vi "sc5511a_spf_select_devices.vi"(5 "error in (no error)":errorcluster) -> (14 "Selected Resource":string, 19 "error out":errorcluster)   [LabVIEW 2010]
panel:
  in  "Cancel Button 2":bool
  in  "OK Button 2":bool
  out "source":string="No Ports  Found."
  in  "Resource Name":u16(ring) items=["COM1"]
  # "Please select a device from the pull-down menu:"
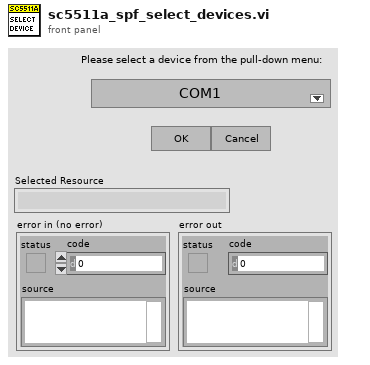
[diagram p1: front panel]
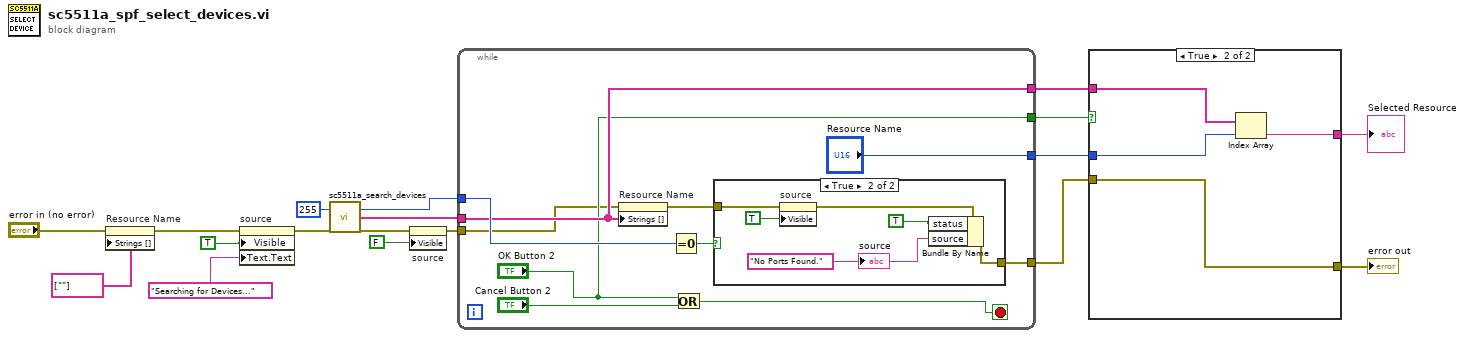
[diagram p0: block diagram]
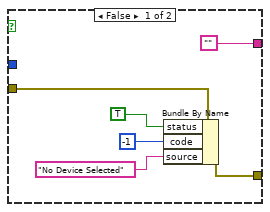
[diagram p2: hidden frame]
diagram:
  n1 = property on="Resource Name" class="Ring (strict)"(error in="error in (no error)", "Strings []"=string[] [""]) -> (error out=w10:errorcluster)  [unwired: 1 in, 1 out]
  n2 = property on="source" class="Str"(error in=w10, "Visible"=TRUE, "Text.Text"="Searching for Devices...") -> (error out=w8:errorcluster)  [unwired: 1 in, 1 out]
  n3 = call "sc5511a_search_devices.vi"("Devices to Search"=u32 255, "error in (no error)"=w8) -> ("Devices Found"=w7:u32, "Port_Name"=w6:string[], "error out"=w4:errorcluster)  [unwired: 15 in]
  n4 = property on="source" class="Str"(error in=w4, "Visible"=FALSE) -> (error out=w3:errorcluster)  [unwired: 1 in, 1 out]
  n5 = while {
    tunnel: ["Resource Name"] -> w17
    tunnel: [w22] -> w18
    tunnel: ["OK Button 2"] -> w16
    tunnel: w3 -> [w19]
    tunnel: [w25] -> w12
    tunnel: w7 -> [w23]
    tunnel: w6 -> [w22]
    stop <- w24 stop-if-true
    n6 = property on="Resource Name" class="Ring (strict)"(error in=w19, "Strings []"=w22) -> (error out=w26:errorcluster)  [unwired: 1 in, 1 out]
    n7 = Equal To 0?(x=w23) -> (x = 0?=w27:bool)
    n8 = Or(x="OK Button 2", y="Cancel Button 2") -> (x .or. y?=w24:bool)
    n9 = case shown="True" w27 {
      tunnel: w26 -> [w29 w32]
      tunnel: [w29 w35] -> w25
      frame False {
      }
      frame True {
        w30 = "No Ports Found." ("source")
        n10 = property on="source" class="Str"(error in=w32, "Visible"=TRUE) -> (error out=w33:errorcluster)  [unwired: 1 in, 1 out]
        n11 = Bundle By Name(cluster=w33, "status"=TRUE, "source"=w30) -> (w35:errorcluster)
        "source" <- w30
      }
    }
  }
  n12 = case shown="True" w16 {
    tunnel: w18 -> [_ w45]
    tunnel: w17 -> [_ w44]
    tunnel: ["" w43] -> w15
    tunnel: w12 -> [w40 w42]
    tunnel: [w38 w42] -> w11
    frame False {
      n13 = Bundle By Name(cluster=w40, "status"=TRUE, "code"=-1, "source"="No Device Selected") -> (w38:errorcluster)
    }
    frame True {
      n14 = Index Array(array=w45, index=w44) -> (element=w43:string)
    }
  }
  "Selected Resource" <- w15
  "error out" <- w11
